vi "Delay32Bit.vi"(3 "delay(ticks)":u32, 4 "In":bool) -> (1 "Out":bool)   [LabVIEW 2014]
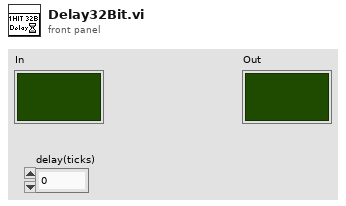
[diagram p1: front panel]
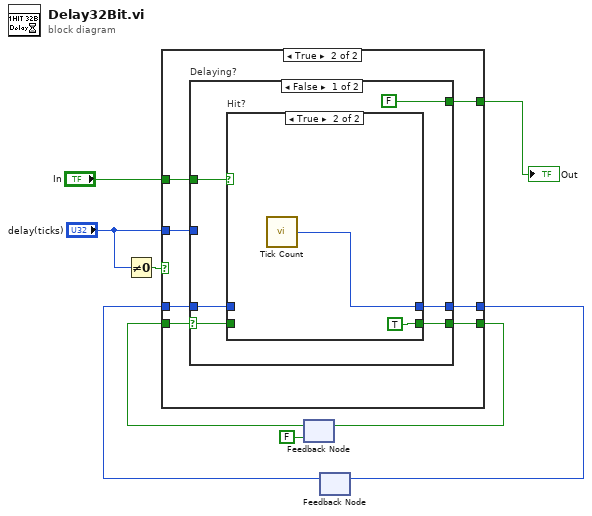
[diagram p0: block diagram]
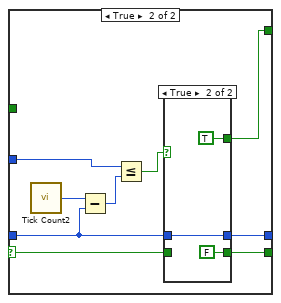
[diagram p4: hidden frame]
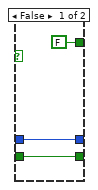
[diagram p5: hidden frame]
diagram:
  n1 = Not Equal To 0?(x="delay(ticks)") -> (x != 0?=w3:bool)
  n2 = feedback #1(FALSE) -> (w1:bool)
  n3 = feedback #2() -> (w7:u32)  [unwired: 1 in]
  n4 = case shown="True" w3 {
    tunnel: "In" -> [w12 w19]
    tunnel: [w11 w18] -> w8
    tunnel: w7 -> [w11 w17]
    tunnel: [w10 w16] -> w6
    tunnel: w1 -> [w10 w15]
    tunnel: [w12 w14] -> w4
    tunnel: "delay(ticks)" -> [_ w13]
    frame False {
    }
    frame True {
      n5 = case "Delaying?" shown="False" w15 {
        selector: w15 -> [w21 w33]
        tunnel: w19 -> [w25 _]
        tunnel: [w24 w30] -> w18
        tunnel: w17 -> [w23 w31]
        tunnel: [w22 w32] -> w16
        tunnel: [FALSE w34] -> w14
        tunnel: w13 -> [_ w38]
        frame False {
          n6 = case "Hit?" shown="True" w25 {
            tunnel: [w27 w29] -> w24
            tunnel: w23 -> [w27 _]
            tunnel: [w26 TRUE] -> w22
            tunnel: w21 -> [w26 _]
            frame False {
            }
            frame True {
              n7 = call "Tick Count"() -> ("Tick Count(Ticks)"=w29:u32)
            }
          }
        }
        frame True {
          n8 = call "Tick Count2"() -> ("Tick Count(Ticks)"=w37:u32)
          n9 = Subtract(x=w37, y=w31) -> (x-y=w36:u32)
          n10 = Less Or Equal?(x=w38, y=w36) -> (x <= y?=w35:bool)
          n11 = case shown="True" w35 {
            tunnel: [FALSE TRUE] -> w34
            tunnel: w33 -> [w40 _]
            tunnel: [w40 FALSE] -> w32
            tunnel: w31 -> [w41 w43]
            tunnel: [w41 w43] -> w30
            frame False {
            }
            frame True {
            }
          }
        }
      }
    }
  }
  "Out" <- w4
  n12 = feedback-in #1(w6) -> ()
  n13 = feedback-in #2(w8) -> ()
